vi "PRIOR_IFilterOpen.vi"(8 "error in (no error)":errorcluster, 11 "Port":i32=5) -> (0 "error out":errorcluster, 3 "PRIORLib Out":T1)   [LabVIEW 2010]
panel:
  in  "PRIORLib.IScan":refnum<k7>
  in  "PRIORLib.IFilterIn":refnum<k7>
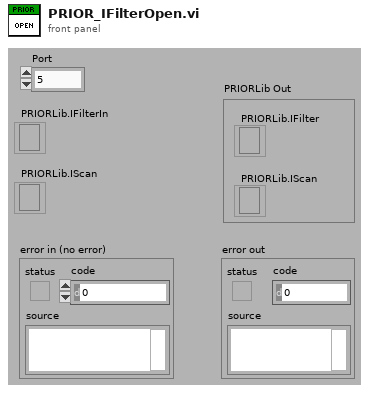
[diagram p1: front panel]
types:
  T1 = cluster{"PRIORLib.IFilter":refnum<k7>, "PRIORLib.IScan":refnum<k7>}
  T2 = cluster{"PRIORLib.IFilterIn":refnum<k7>, "PRIORLib.IScan":refnum<k7>}
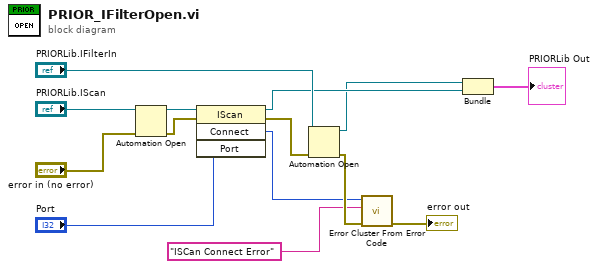
[diagram p0: block diagram]
diagram:
  n1 = Automation Open(error in (no error)="error in (no error)", Automation Refnum="PRIORLib.IScan") -> (Automation Refnum=w12:refnum<k7>, error out=w9:errorcluster)  [unwired: 2 in]
  n2 = invoke class="IScan" method="Connect"(reference=w12, error in=w9, "Port"="Port") -> (reference out=w3:refnum<k7>, error out=w8:errorcluster, "Connect"=w5:i32)  [unwired: 1 in, 1 out]
  n3 = Automation Open(error in (no error)=w8, Automation Refnum="PRIORLib.IFilterIn") -> (Automation Refnum=w2:refnum<k7>, error out=w7:errorcluster)  [unwired: 2 in]
  n4 = call <vilib>:"Error Cluster From Error Code.vi"("error in (no error)"=w7, "error message (\"\")"="ISCan Connect Error" ("error message (\"\")"), "error code (0)"=w5) -> ("error out"=→"error out":errorcluster)  [unwired: 6 in]
  n5 = Bundle("PRIORLib.IFilterIn"=w2, "PRIORLib.IScan"=w3) -> (→"PRIORLib Out":T2)  [unwired: 1 in]
